vi "603xA Set Soft Limits.vi"(8 "error in (no error)":errorcluster, 9 "current limit (0A)":dbl format="%.4f", 10 "voltage limit (0V)":dbl format="%.4f", 11 "VISA resource name":refnum<visa-resource-name>) -> (0 "error out":errorcluster, 3 "VISA resource name out":refnum<visa-resource-name>)   [LabVIEW 2020, in "Agilent 6XXX Series.lvlib"]
doc: "This function sets the upper limits on the voltage and current programming values that the power supply will accept. This function is valid for the HP603XA series only."
uses:
  <instrlib>/Agilent 6XXX Series/Agilent 6XXX Series.lvlib
panel:
  # "HP603XA series only"
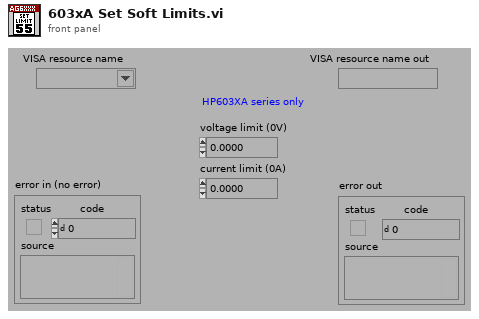
[diagram p1: front panel]
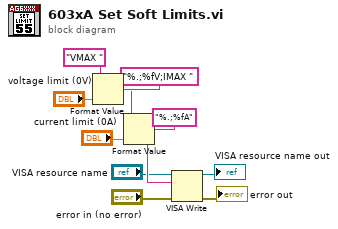
[diagram p0: block diagram]
diagram:
  n1 = Format Value(string ("")="VMAX ", format string="%.;%fV;IMAX ", value (0)="voltage limit (0V)") -> (output string=w6:string)
  n2 = Format Value(string ("")=w6, format string="%.;%fA", value (0)="current limit (0A)") -> (output string=w5:string)
  n3 = VISA Write(VISA resource name="VISA resource name", write buffer=w5, error in (no error)="error in (no error)") -> (VISA resource name out=→"VISA resource name out":refnum<visa-resource-name>, error out=→"error out":errorcluster)  [unwired: 1 out]
